vi "Destroy.vi"(8 "error in (no error)":errorcluster, 11 "response in":refnum<class "response.lvclass">) -> (0 "error out":errorcluster)   [LabVIEW 2020, in "http.lvlib" / "response.lvclass"]
uses:
  response.lvclass
  response.lvclass/response.ctl
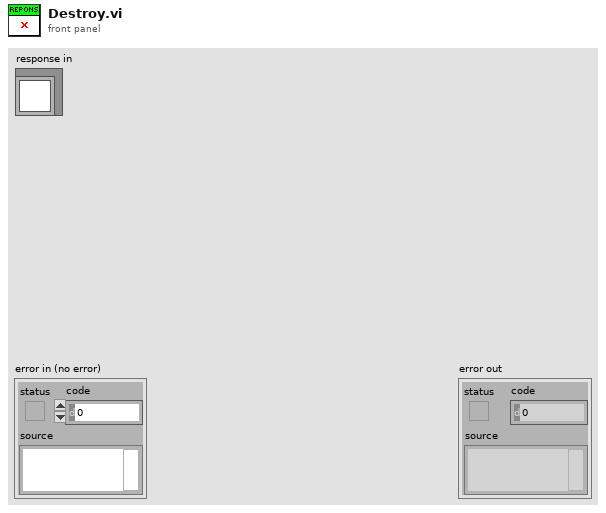
[diagram p1: front panel]
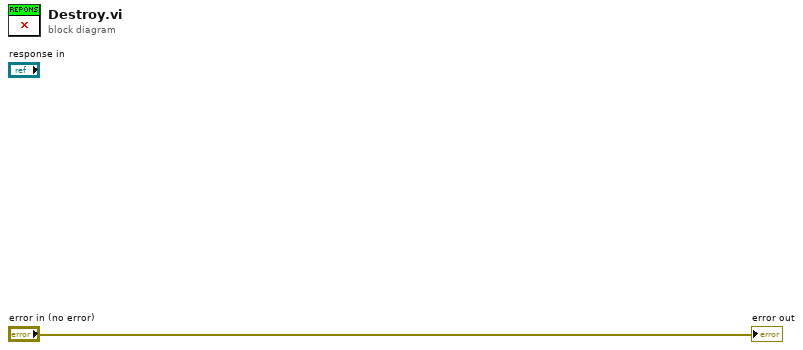
[diagram p0: block diagram]
diagram:
  "error out" <- "error in (no error)"
